vi "LINX - PWM N Channel.vi"() -> ()   [LabVIEW 2019]
doc: "This example demonstrates how to generate N Channels of PWM output using a LINX device."
uses:
  <vilib>/MakerHub/LINX/Public/Peripherals/Digital/Digital Read 1 Chan.vi
  <vilib>/MakerHub/LINX/Public/Peripherals/Digital/Digital Read N Chans.vi
  <vilib>/MakerHub/LINX/Private/Local IO/LinxDigitalRead.vi
  <vilib>/MakerHub/LINX/Public/Utilities/Check Channel.vi
  <vilib>/MakerHub/LINX/Public/Utilities/Open Serial.vi
  <vilib>/MakerHub/LINX/Public/Peripherals/PWM/PWM Set Duty Cycle N Chans.vi
  <vilib>/MakerHub/LINX/Private/Utilties/Generate Error.vi
  <vilib>/MakerHub/LINX/LMH-LINX.lvlib
panel:
  out "Boolean":bool
  in  "PWM Channels":u8[](array[numeric])=[3, 5, 6]
  in  "Duty Cycles":dbl[](array[slide]) min=0.0 max=255.0 step=1.0 scale=0.0..255.0
  in  "Stop Button":bool
  in  "Serial Port":refnum<visa-resource-name>
  # "LINX Device Settings"
  # "PWM Duty Cycles"
  # "PWM N Channel Example\n\nThis example demonstrates how to set the dutry cycle of multiple PWM channels.\nA duty cycle of 0 coresponds to 0% on and a duty cycle of 1 coresponds to 100% on.\n\nInstructions\n1. Select the COM Port associated with the LINX Device.\n2. Select the PWM Channels to write to.\n3. Click the Run Arrow."
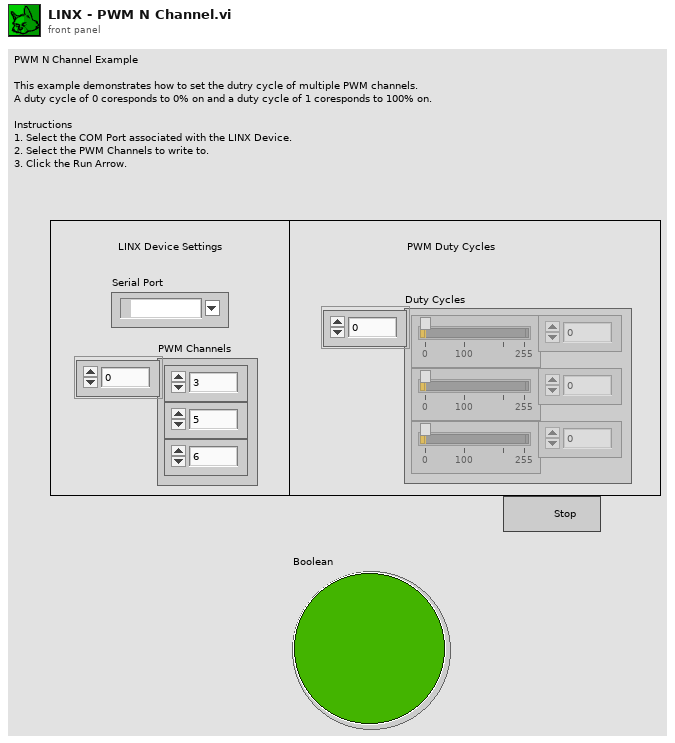
[diagram p1: front panel]
types:
  T1 = typedef "LMH-LINX.lvlib/LINX Ref.ctl" = cluster{"IO":T2, "Interface":T3, "LINX Device Config":T4}
  T2 = typedef "LMH-LINX.lvlib/Platform.ctl" = enum16{"Remote", "Local"}
  T3 = typedef "LMH-LINX.lvlib/Interface.ctl" = enum16{"Serial", "TCP"}
  T4 = typedef "LMH-LINX.lvlib/Device.lvlib/LINX Device Config.ctl" = cluster{"Interface":T3, "COM Port":refnum<visa-resource-name>, "TCP Configuration":T5, "Device Family":u8, "Device ID":u8, "Device Name":string, "TCP Ref":refnum<k5>, "Channels":T6}
  T5 = typedef "LMH-LINX.lvlib/Device.lvlib/TCP Config.ctl" = cluster{"IP Address":string, "Port":u16}
  T6 = typedef "LMH-LINX.lvlib/Channels.ctl" = cluster{"DI":u8[], "DO":u8[], "AI":u8[], "AO":u8[], "PWM":u8[], "QE":u8[], "UART":u8[], "I2C 2":u8[], "SPI":u8[], "CAN":u8[], "Servo":u8[], "AI Ref (V)":dbl, "AI Resolution (Bits)":u8, "AO Ref (V)":dbl, "AO Resolution (Bits)":u8}
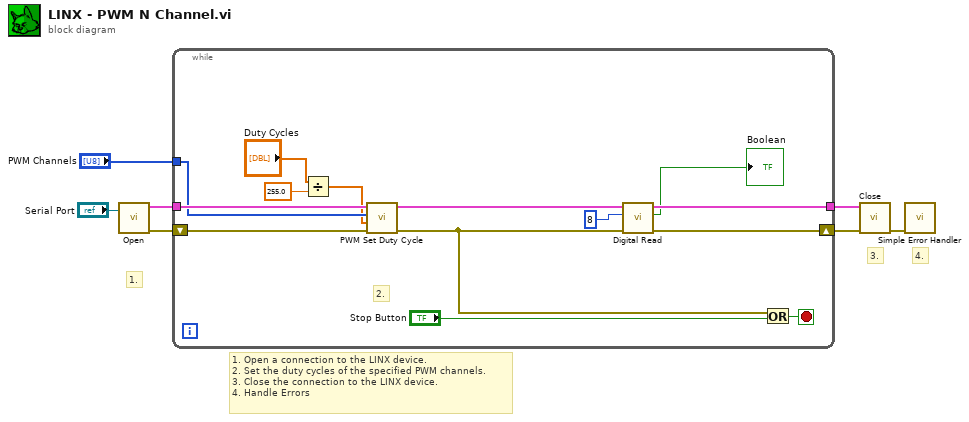
[diagram p0: block diagram]
diagram:
  # "1. Open a connection to the LINX device.\n2. Set the duty cycles of the specified PWM channels.\n3. Close the connection to the LINX device.\n4. Handle Errors"
  # "4."
  # "3."
  # "1."
  n1 = call-poly <vilib>:"Open.vi"("Serial Port"="Serial Port") -> ("Error Out"=w6:errorcluster, "LINX Resource"=w7:T1)  [unwired: 8 in, 1 out]
  n2 = while {
    tunnel: w7 -> [w18]
    tunnel: [w11] -> w5
    shift-right: [w12] -> w4
    shift-left: w6 -> [w19]
    tunnel: "PWM Channels" -> [w17]
    stop <- w21 stop-if-true
    # "2."
    n3 = Divide(x="Duty Cycles", y=255.0) -> (x/y=w14:dbl[])
    n4 = call-poly <vilib>:"PWM Set Duty Cycle.vi"("Error In"=w19, "Duty Cycles"=w14, "PWM Channels"=w17, "LINX Resource"=w18) -> ("Error Out"=w13:errorcluster, "LINX Resource"=w10:T1)  [unwired: 6 in]
    n5 = call-poly <vilib>:"Digital Read.vi"("Error In"=w13, "DI Channel"=u8 8, "LINX Resource"=w10) -> ("Error Out"=w12:errorcluster, "DI Value"=→"Boolean":bool, "LINX Resource"=w11:T1)  [unwired: 6 in]
    n6 = Or(x=w13, y="Stop Button") -> (x .or. y?=w21:bool)
  }
  n7 = call <vilib>:"Close.vi"("Error In"=w4, "LINX Resource"=w5) -> ("Error Out"=w2:errorcluster)  [unwired: 9 in]
  n8 = call <vilib>:"Simple Error Handler.vi"("error in (no error)"=w2) -> ()  [unwired: 4 in, 5 out]
